vi "rollingArray (SubVI).vi"(10 "new element/subarray":dbl, 11 "array":dbl[](array[numeric])) -> (3 "Array":dbl[](array[numeric]))   [LabVIEW 2014]
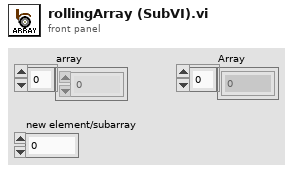
[diagram p1: front panel]
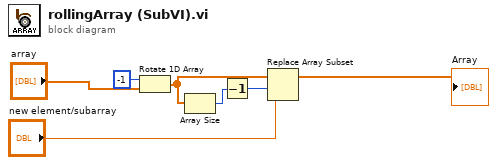
[diagram p0: block diagram]
diagram:
  n1 = Rotate 1D Array(1:"array", 2:-1 ("n")) -> (0:w2:dbl[])
  n2 = Array Size(array=w2) -> (size(s)=w3:i32)
  n3 = Decrement(x=w3) -> (x-1=w4:i32)
  n4 = Replace Array Subset(array=w2, new element="new element/subarray", index=w4) -> (→"Array":dbl[])
